vi "Temp Control Set Temp.vi"(8 "error in (no error)":errorcluster, 10 "Temp C":dbl, 11 "Application in":refnum<class "Application.lvclass">) -> (0 "error out":errorcluster, 3 "Application out":refnum<class "Application.lvclass">)   [LabVIEW 2023, in "Application.lvlib" / "Application.lvclass"]
uses:
  Application.lvclass
  Application.lvclass/Application.ctl
  Hardware/Temperature Controller Messages/Set Temp Msg/Set Temp Msg.lvclass
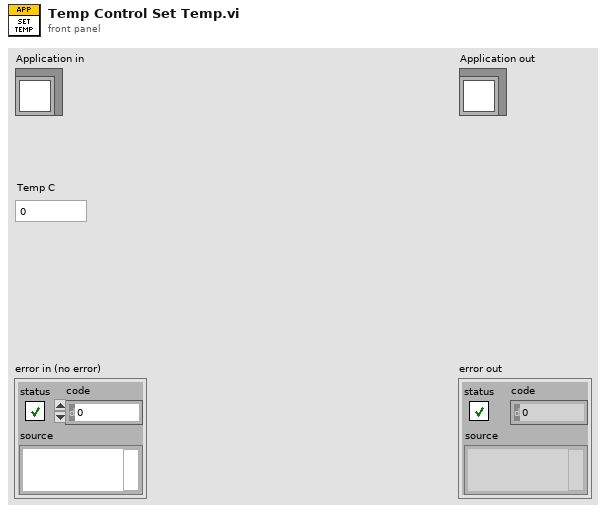
[diagram p1: front panel]
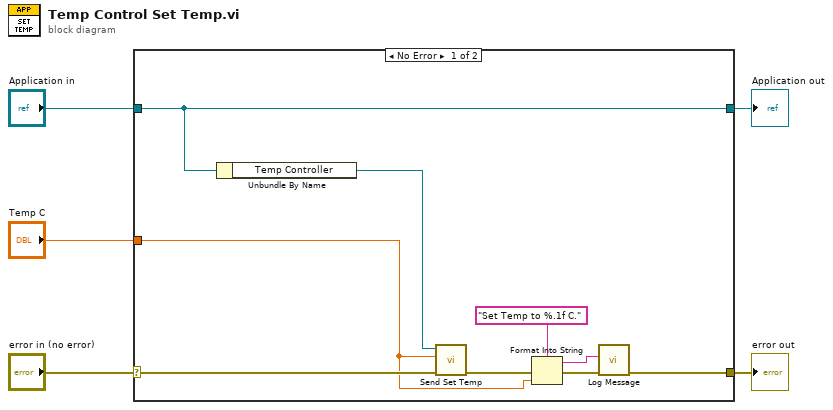
[diagram p0: block diagram]
diagram:
  n1 = case shown="No Error" "error in (no error)" {
    selector: "error in (no error)" -> [w12 w16]
    tunnel: [w11 w16] -> w4
    tunnel: [w14 w15] -> w2
    tunnel: "Application in" -> [w14 w15]
    tunnel: "Temp C" -> [w7 _]
    frame No Error {
      n2 = Unbundle By Name(w14) -> ("Temp Controller"=w13:refnum<class "Message Enqueuer.lvclass">)
      n3 = call "Send Set Temp.vi"("error in (no error)"=w12, "Temp C"=w7, "Message Enqueuer"=w13) -> ("error out"=w9:errorcluster)  [unwired: 7 in, 1 out]
      n4 = Format Into String(format string="Set Temp to %.1f C.", error in=w9, w7) -> (resulting string=w10:string, error out=w8:errorcluster)  [unwired: 1 in]
      n5 = call "Log Message.vi"("error constant"=w8, "input"=w10) -> ("error constant 2"=w11:errorcluster)  [unwired: 8 in, 1 out]
    }
    frame Error {
    }
  }
  "error out" <- w4
  "Application out" <- w2
